vi "PicoScopeospaIsReady.vi"(8 "error in (no error)":errorcluster, 11 "handle in":i16) -> (0 "error out":errorcluster, 3 "handle out":i16, 6 "ready":i16=1)   [LabVIEW 2024]
doc: "Calls IsReady"
uses:
  psospa.dll
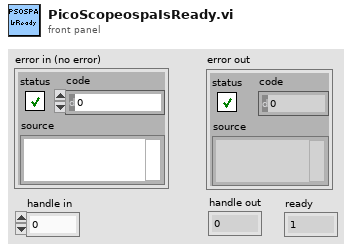
[diagram p1: front panel]
types:
  T1 = cluster{"status":bool, "code":u32, "source":string}
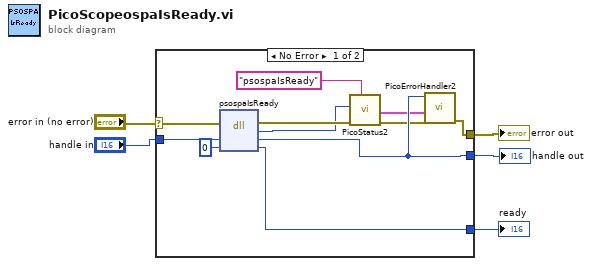
[diagram p0: block diagram]
diagram:
  n1 = case shown="No Error" "error in (no error)" {
    selector: "error in (no error)" -> [w15 w17]
    tunnel: "handle in" -> [w16 w18]
    tunnel: [w12 w18] -> w5
    tunnel: [w7 w17] -> w4
    tunnel: [w9 _] -> w3
    frame No Error {
      n2 = dll-call lib="F:/Picoscope3000e/Scope_LabView/ps3000e/Treiber_und_SubVis/psospa.dll" fn="psospaIsReady" ("ps3000.dll:_ps3000_open_unit@0")(error in=w15, "handle"=w16, "ready"=i16 0) -> (error out=w14:errorcluster, "PICO_STATUS"=w10:u32, "handle"=w12:i16, "ready"=w9:i16)  [unwired: 2 in, 1 out]
      n3 = call "PicoStatus2.vi"("PICO source"="psospaIsReady" ("source"), "Error in"=w14, "PICO STATUS"=w10) -> ("error out"=w8:errorcluster, "PICO_STATUS out"=w6:T1)  [unwired: 5 in]
      n4 = call "PicoErrorHandler2.vi"("error in (no error)"=w8, "PICO_STATUS in"=w6, "handle In"=w12) -> ("error out"=w7:errorcluster)  [unwired: 8 in]
    }
    frame Error {
    }
  }
  "error out" <- w4
  "handle out" <- w5
  "ready" <- w3
